vi "Acquire and save Single Image.vi"(4 "Save image?":bool, 5 "File Path":path, 8 "Camera Name":refnum<k21> caption="IMAQdx Session") -> (0 "error out":errorcluster, 3 "Image":T1(plugin-control))   [LabVIEW 2018]
doc: "The Acquire Single Image (Snap) example acquires an image and displays the image in an image control. A snap is appropriate for low-speed or single-capture applications in which ease of programming is essential."
uses:
  <vilib>/vision/driver/NI_Vision_Acquisition_Software.lvlib
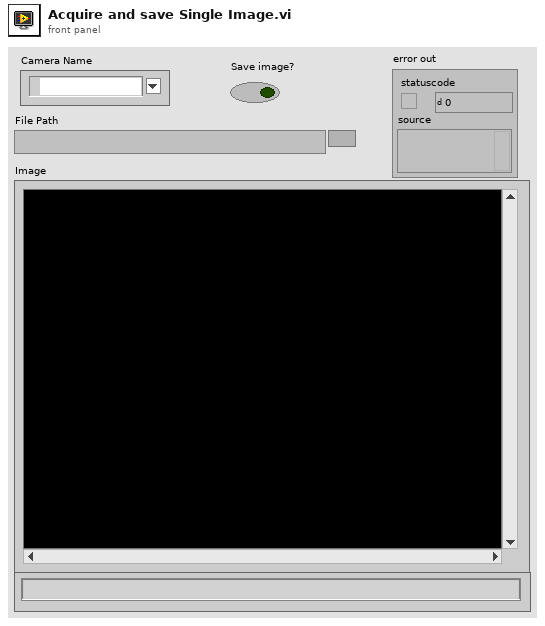
[diagram p1: front panel]
types:
  T1 = typedef "IMAQ Image.ctl" = refnum<image>
  T2 = typedef "IMAQdx.ctl" = refnum<k21>
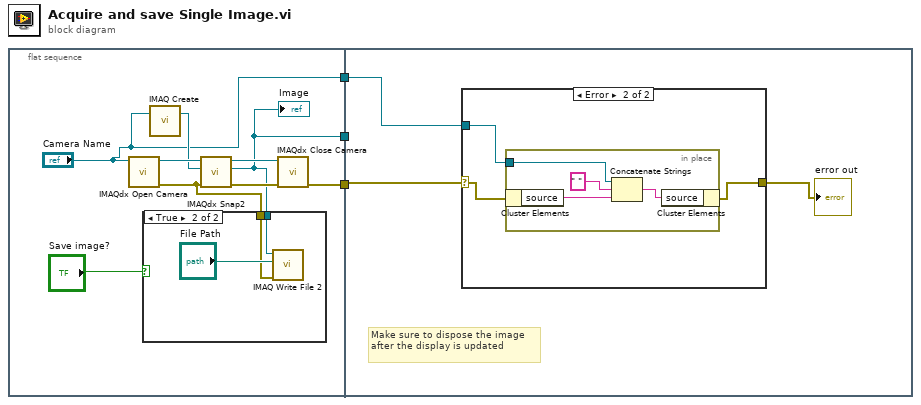
[diagram p0: block diagram]
diagram:
  n1 = flat-sequence {
    tunnel: [w11] -> w3
    tunnel: [w7] -> w2
    tunnel: ["Camera Name"] -> w1
    tunnel: w3 -> [w16]
    tunnel: w2 -> [_]
    tunnel: w1 -> [w17]
    frame #0 {
      n2 = call <vilib>:"IMAQdx Open Camera.vi"("Session In"="Camera Name") -> ("error out"=w6:errorcluster, "Session Out"=w10:T2)  [unwired: 2 in, 7 out]
      n3 = call "IMAQ Create"("Image Name"="Camera Name") -> ("New Image"=w8:T1)  [unwired: 3 in, 2 out]
      n4 = call <vilib>:"IMAQdx Snap2.vi"("error in"=w6, "Image In"=w8, "Session In"=w10) -> ("error out"=w9:errorcluster, "Image Out"=w7:T1, "Session Out"=w12:T2)  [unwired: 6 in]
      "Image" <- w7
      n5 = case shown="True" "Save image?" {
        tunnel: w7 -> [_ w15]
        tunnel: w6 -> [_ w13]
        frame False {
        }
        frame True {
          n6 = call-poly "IMAQ Write File 2"("error in (no error)"=w13, "File Path"="File Path", "Image"=w15) -> ()  [unwired: 7 in, 2 out]
        }
      }
      n7 = call <vilib>:"IMAQdx Close Camera.vi"("error in"=w9, "Session In"=w12) -> ("error out"=w11:errorcluster)  [unwired: 9 out]
    }
    frame #1 {
      # "Make sure to dispose the image after the display is updated"
      n8 = case shown="Error" w16 {
        selector: w16 -> [w19 w22]
        tunnel: [w19 w20] -> w18
        tunnel: w17 -> [_ w21]
        frame No Error {
        }
        frame Error {
          n9 = in-place {
            in-place-border: w21 -> [w24]
            n10 = in-place-cluster #1(w22) -> ("source"=w26:string)
            n11 = Concatenate Strings(w24, " " ("string"), w26) -> (w23:string)
            n12 = in-place-cluster #1("source"=w23) -> (w20:errorcluster)
          }
        }
      }
      "error out" <- w18
    }
  }
